vi "Glyph Transform Client.vi"(8 "error in (no error)":errorcluster, 10 "Transform":T1, 11 "glyph ref in":i64) -> (0 "error out":errorcluster, 3 "glyph ref out":i64)   [LabVIEW 2023, in "Freetype Drawer.lvlib"]
uses:
  Freetype Drawer.lvlib
  <vilib>/Analysis/Matrix/Datatypes/RealMatrix.ctl
  <vilib>/Analysis/Matrix/NI_Matrix.lvlib
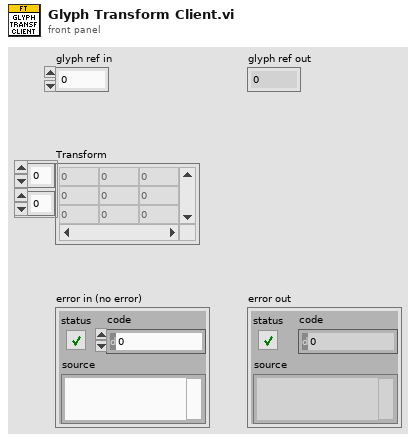
[diagram p1: front panel]
types:
  T1 = typedef "NI_Matrix.lvlib/RealMatrix.ctl" = dbl[][]
  T2 = typedef "Freetype Drawer.lvlib/Outline Glyph Rec.ctl" = cluster{"root":T3, "Outline":cluster{"n_contours":i16, "n_points":i16, "points ref":i64, "tags ref":i64, "contours ref":i64, "flags":i32}}
  T3 = typedef "Freetype Drawer.lvlib/Glyph Rec.ctl" = cluster{"library ref":i64, "class ref":i64, "format":i32, "advance":cluster{"x":i32, "y":i32}}
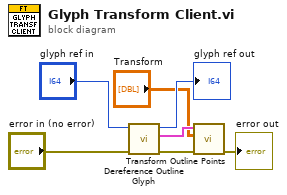
[diagram p0: block diagram]
diagram:
  n1 = call "Dereference Outline Glyph.vi"("error in (no error)"="error in (no error)", "glyph ref in"="glyph ref in") -> ("error out"=w6:errorcluster, "Outline Glyph Rec"=w5:T2, "glyph ref out"=→"glyph ref out":i64)  [unwired: 7 in]
  n2 = call "Transform Outline Points.vi"("error in (no error)"=w6, "2xN Matrix"="Transform", "Outline Glyph Rec"=w5) -> ("error out"=→"error out":errorcluster)  [unwired: 7 in, 1 out]
